vi "Demo.vi"() -> ()   [LabVIEW 2015]
uses:
  KDemoBase Class/KDemoBase.lvclass
  KDemoDerived Class/KDemoDerived.lvclass
  KDemo XControl/KDemo.xctl
  KDemoDerived Class/KDemoDerived.lvclass/KDemoDerived.ctl
  KDemoBase Class/KDemoBase.lvclass/KDemoBase.ctl
  KDemoDerived Class/Write String.vi
  KDemoBase Class/Write Value.vi
  KDemoDerived Class/Write Integer.vi
  KDemoBase Class/Write Boolean.vi
  KDemoBase Class/Read Value.vi
  KDemoDerived Class/Read String.vi
  KDemoBase Class/Read Boolean.vi
  KDemoDerived Class/Read Integer.vi
panel:
  out "KDemo 2":refnum<class "KDemoBase.lvclass">(xcontrol)
  out "Base: Boolean":bool
  in  "KDemo":refnum<class "KDemoBase.lvclass">(xcontrol)
  out "Array2: Integer":i32
  out "Derived: Integer":i32
  out "Array2: Boolean":bool
  out "Array2: String":string
  out "Array2: Value":dbl
  out "Array1: Value":dbl
  out "Array length":i32
  out "Base2: String":string
  out "Derived: String":string
  out "Derived: Value":dbl
  out "Base: Value":dbl
  out "Base2: Value":dbl
  in  "Cluster":T1
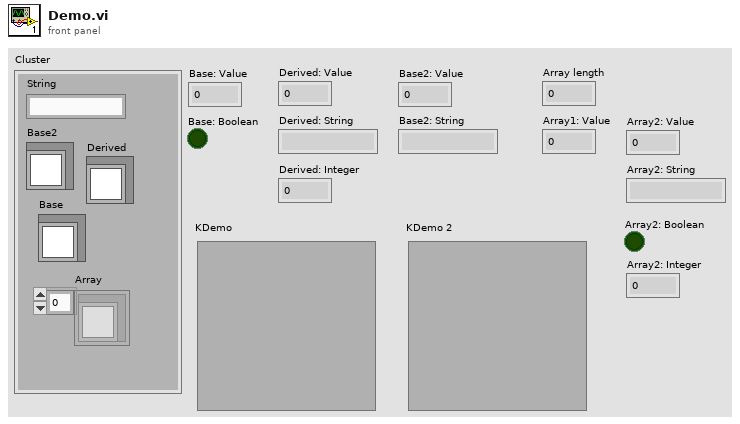
[diagram p1: front panel]
types:
  T1 = cluster{"String":string, "Base":refnum<class "KDemoBase.lvclass">, "Derived":refnum<class "KDemoDerived.lvclass">, "Base2":refnum<class "KDemoBase.lvclass">, "Array":refnum<class "KDemoBase.lvclass">[]}
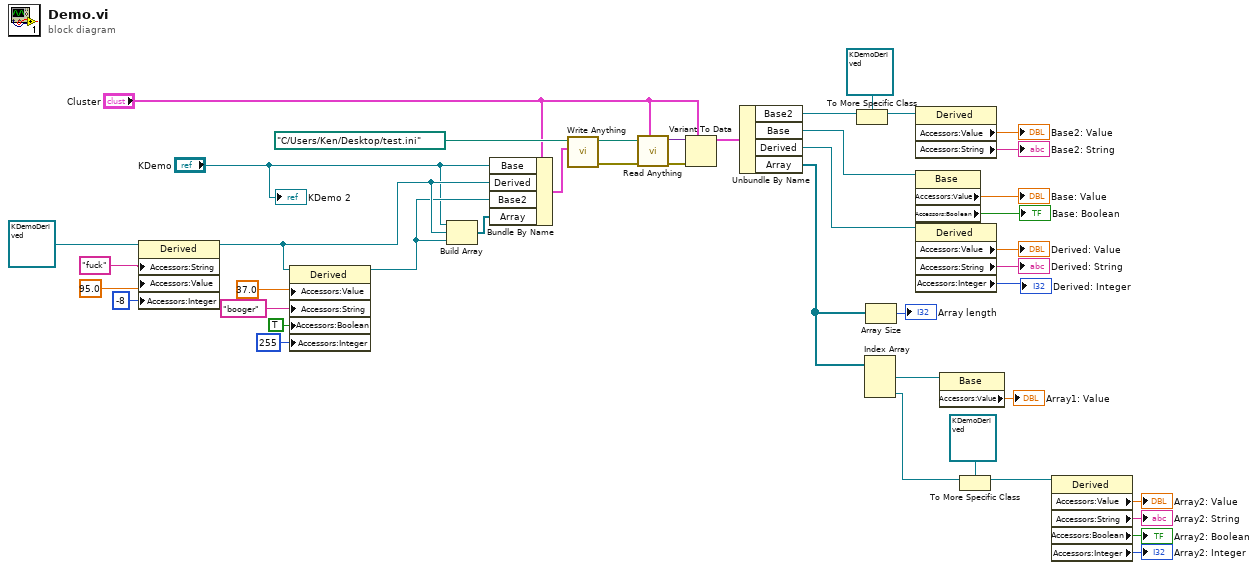
[diagram p0: block diagram]
diagram:
  n1 = property class="Derived"(reference=refnum<class "KDemoDerived.lvclass"> refnum ("Gen2"), "Accessors:String"="fuck" ("String"), "Accessors:Value"=95.0 ("Numeric"), "Accessors:Integer"=-8 ("Integer")) -> (reference out=w36:refnum<class "KDemoDerived.lvclass">)  [unwired: 1 in, 1 out]
  n2 = property class="Derived"(reference=w36, "Accessors:Value"=37.0 ("Numeric"), "Accessors:String"="booger" ("String"), "Accessors:Boolean"=TRUE ("Boolean"), "Accessors:Integer"=255 ("Integer")) -> (reference out=w2:refnum<class "KDemoDerived.lvclass">)  [unwired: 1 in, 1 out]
  n3 = Build Array("KDemo", w36, w2) -> (w33:refnum<class "KDemoBase.lvclass">[])
  n4 = Bundle By Name(cluster="Cluster", "Base"="KDemo", "Derived"=w36, "Base2"=w2, "Array"=w33) -> (w15:T1)
  n5 = call "Write Anything.vi"("Anything"=w15, "Path (dialog)"=path "C:/Users/Ken/Desktop/test.ini") -> ("Error Out"=w42:errorcluster, "Path out"=w35:path)  [unwired: 8 in]
  n6 = call "Read Anything.vi"("Type of Anything"="Cluster", "Error In"=w42, "Path (dialog)"=w35) -> ("Error Out"=w32:errorcluster, "Anything"=w31:variant)  [unwired: 6 in, 1 out]
  n7 = Variant To Data(error in=w32, type="Cluster", Variant=w31) -> (data=w34:T1)  [unwired: 1 out]
  n8 = Unbundle By Name(w34) -> ("Base2"=w20:refnum<class "KDemoBase.lvclass">, "Base"=w25:refnum<class "KDemoBase.lvclass">, "Derived"=w23:refnum<class "KDemoDerived.lvclass">, "Array"=w29:refnum<class "KDemoBase.lvclass">[])
  n9 = To More Specific Class(target class=refnum<class "KDemoDerived.lvclass"> refnum ("Gen2"), reference=w20) -> (specific class reference=w18:refnum<class "KDemoDerived.lvclass">)  [unwired: 1 in, 1 out]
  n10 = Index Array(array=w29) -> (element #1=w27:refnum<class "KDemoBase.lvclass">, element #3=w26:refnum<class "KDemoBase.lvclass">)  [unwired: 3 in, 1 out]
  n11 = Array Size(array=w29) -> (size(s)=→"Array length":i32)
  n12 = property class="Derived"(reference=w18) -> ("Accessors:Value"=→"Base2: Value":dbl, "Accessors:String"=→"Base2: String":string)  [unwired: 1 in, 2 out]
  n13 = property class="Base"(reference=w25) -> ("Accessors:Value"=→"Base: Value":dbl, "Accessors:Boolean"=→"Base: Boolean":bool)  [unwired: 1 in, 2 out]
  n14 = property class="Derived"(reference=w23) -> ("Accessors:Value"=→"Derived: Value":dbl, "Accessors:String"=→"Derived: String":string, "Accessors:Integer"=→"Derived: Integer":i32)  [unwired: 1 in, 2 out]
  n15 = property class="Base"(reference=w27) -> ("Accessors:Value"=→"Array1: Value":dbl)  [unwired: 1 in, 2 out]
  n16 = To More Specific Class(target class=refnum<class "KDemoDerived.lvclass"> refnum ("Gen2"), reference=w26) -> (specific class reference=w10:refnum<class "KDemoDerived.lvclass">)  [unwired: 1 in, 1 out]
  n17 = property class="Derived"(reference=w10) -> ("Accessors:Value"=→"Array2: Value":dbl, "Accessors:String"=→"Array2: String":string, "Accessors:Boolean"=→"Array2: Boolean":bool, "Accessors:Integer"=→"Array2: Integer":i32)  [unwired: 1 in, 2 out]
  "KDemo 2" <- "KDemo"
